vi "Create Video Filename.vi"(8 "error in (no error)":errorcluster, 11 "SB App in":refnum<class "SB App.lvclass">) -> (0 "error out":errorcluster, 2 "Video Filename":string, 3 "SB App out":refnum<class "SB App.lvclass">)   [LabVIEW 2020, in "SB App.lvlib" / "SB App.lvclass"]
uses:
  SB App.lvclass
  SB App.lvclass/SB App.ctl
  <vilib>/regexp/Match Regular Expression.xnode
  SquareBattle/Team/Team.lvclass
  SquareBattle/Game/Game.lvclass
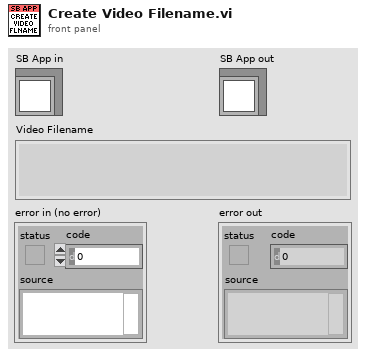
[diagram p1: front panel]
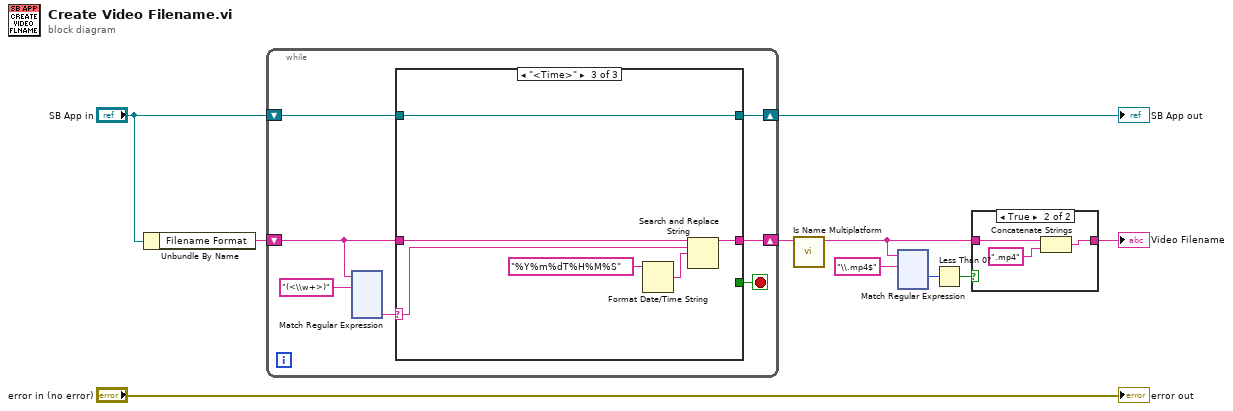
[diagram p0: block diagram]
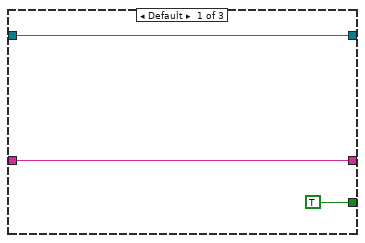
[diagram p2: hidden frame]
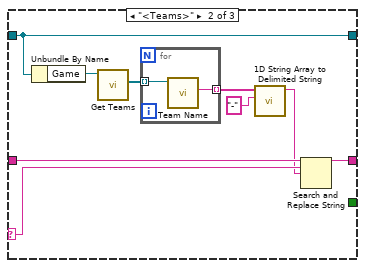
[diagram p3: hidden frame]
diagram:
  n1 = Unbundle By Name("SB App in") -> ("Filename Format"=w1:string)
  n2 = while {
    shift-right: [w11] -> w3
    shift-left: w1 -> [w15]
    shift-right: [w13] -> w9
    shift-left: "SB App in" -> [w14]
    stop <- w12 stop-if-true
    n3 = xnode "Match Regular Expression"("input string"=w15, "regular expression"="(<\\w+>)") -> ("submatch 1"=w16:string)  [unwired: 4 in, 5 out]
    n4 = case shown="\"<Time>\"" w16 {
      selector: w16 -> [_ w23 w34]
      tunnel: w15 -> [w19 w24 w36]
      tunnel: w14 -> [w18 w27 w37]
      tunnel: [w18 w27 w37] -> w13
      tunnel: [TRUE _ _] -> w12
      tunnel: [w19 w21 w35] -> w11
      frame Default {
      }
      frame "<Teams>" {
        n5 = Unbundle By Name(w27) -> ("Game"=w29:refnum<class "Game.lvclass">)
        n6 = call "Get Teams.vi"("Game in"=w29) -> ("Teams"=w28:refnum<class "Team.lvclass">[])  [unwired: 8 in, 2 out]
        n7 = for {
          tunnel: w28 -> [w31] mode=indexing
          tunnel: [w30] -> w26 mode=indexing
          n8 = call-dynamic "Team Name.vi"("Team in"=w31) -> ("Team Name"=w30:string)  [unwired: 10 in]
        }
        n9 = call <vilib>:"1D String Array to Delimited String.vi"("delimiter"="-", "string array"=w26) -> ("delimited string"=w22:string)  [unwired: 9 in]
        n10 = Search and Replace String(input string=w24, search string=w23, replace string=w22) -> (result string=w21:string)  [unwired: 5 in, 3 out]
      }
      frame "<Time>" {
        n11 = Format Date/Time String(time format string (%c)="%Y%m%dT%H%M%S") -> (date/time string=w33:string)  [unwired: 2 in]
        n12 = Search and Replace String(input string=w36, search string=w34, replace string=w33) -> (result string=w35:string)  [unwired: 5 in, 3 out]
      }
    }
  }
  "SB App out" <- w9
  n13 = call <vilib>:"Is Name Multiplatform.vi"("filename"=w3) -> ("suggested filename"=w2:string)  [unwired: 6 in, 4 out]
  n14 = xnode "Match Regular Expression"("input string"=w2, "regular expression"="\\.mp4$") -> ("offset past match"=w6:i32)  [unwired: 4 in, 4 out]
  n15 = Less Than 0?(x=w6) -> (x < 0?=w5:bool)
  n16 = case shown="True" w5 {
    tunnel: w2 -> [w154 w157]
    tunnel: [w154 w155] -> w4
    frame False {
    }
    frame True {
      n17 = Concatenate Strings(w157, ".mp4" ("string")) -> (w155:string)
    }
  }
  "Video Filename" <- w4
  "error out" <- "error in (no error)"
